vi "check_save_file_valid.vi"(8 "error in":errorcluster, 11 "save file path":path) -> (0 "error out":errorcluster, 3 "valid?":bool)   [LabVIEW 2024]
uses:
  <vilib>/Utility/config.llb/NI_LVConfig.lvlib
  <vilib>/Utility/config.llb/Read Key (U32).vi
  <vilib>/Utility/config.llb/Read Key (String).vi
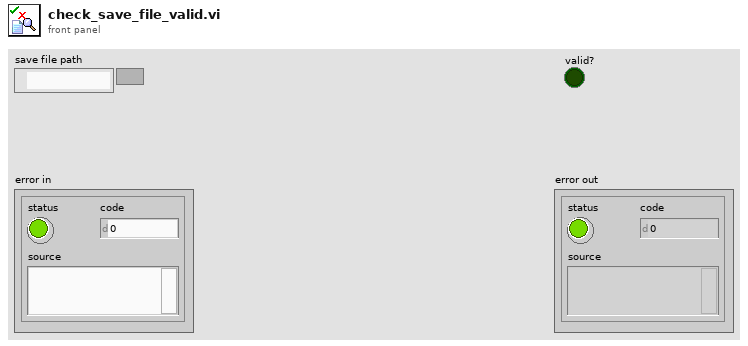
[diagram p1: front panel]
types:
  T1 = typedef "NI_LVConfig.lvlib/Config Data RefNum.ctl" = refnum<k1>
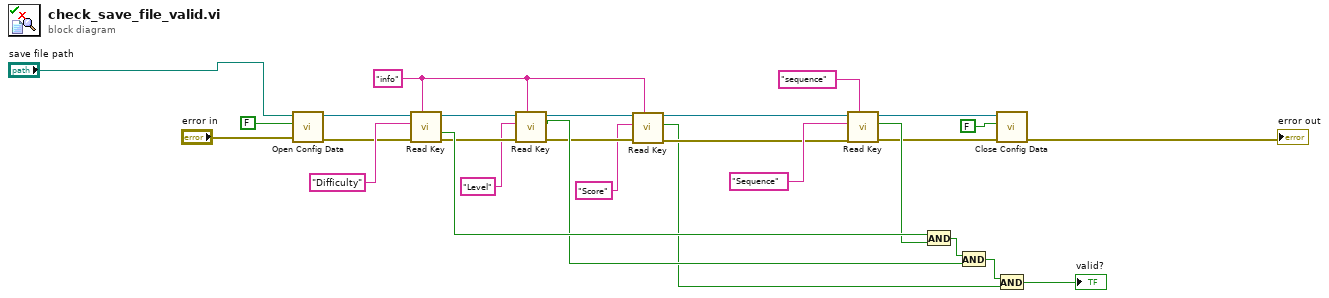
[diagram p0: block diagram]
diagram:
  w10 = "info" ("section")
  n1 = call <vilib>:"Open Config Data.vi"("error in (no error)"="error in", "create file if necessary (T)"=FALSE, "configuration file path"="save file path") -> ("error out"=w21:errorcluster, "refnum"=w27:T1)  [unwired: 6 in, 1 out]
  n2 = call-poly <vilib>:"Read Key.vi"("section"=w10, "error in (no error)"=w21, "key"="Difficulty", "refnum"=w27) -> ("error out"=w19:errorcluster, "found?"=w25:bool, "refnum out"=w20:T1)  [unwired: 4 in, 1 out]
  n3 = call-poly <vilib>:"Read Key.vi"("section"=w10, "error in (no error)"=w19, "key"="Level", "refnum"=w20) -> ("error out"=w12:errorcluster, "found?"=w16:bool, "refnum out"=w11:T1)  [unwired: 4 in, 1 out]
  n4 = call-poly <vilib>:"Read Key.vi"("section"=w10, "error in (no error)"=w12, "key"="Score", "refnum"=w11) -> ("error out"=w8:errorcluster, "found?"=w5:bool, "refnum out"=w7:T1)  [unwired: 4 in, 1 out]
  n5 = call-poly <vilib>:"Read Key.vi"("section"="sequence", "error in (no error)"=w8, "key"="Sequence", "refnum"=w7) -> ("error out"=w15:errorcluster, "found?"=w22:bool, "refnum out"=w14:T1)  [unwired: 4 in, 1 out]
  n6 = And(x=w25, y=w22) -> (x .and. y?=w17:bool)
  n7 = And(x=w17, y=w16) -> (x .and. y?=w6:bool)
  n8 = call <vilib>:"Close Config Data.vi"("error in (no error)"=w15, "write file if changed (T)"=FALSE, "refnum"=w14) -> ("error out"=→"error out":errorcluster)  [unwired: 7 in, 1 out]
  n9 = And(x=w6, y=w5) -> (x .and. y?=→"valid?":bool)
